vi "Programmed Temperature for Step N.vi"(11 "步骤编号":i32) -> (1 "新的温度消息":string, 3 "待维持的温度":dbl)   [LabVIEW 2015, in "Programmatic Controller.lvclass"]
doc: "给定步骤编号，返回该步骤待维持的温度（数值和字符串）。"
uses:
  Programmatic Controller.lvclass
panel:
  in  "新的待维持温度消息":string="新的待维持温度：%d"
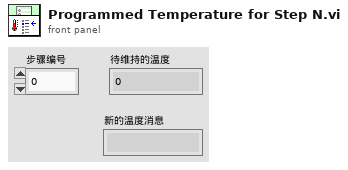
[diagram p1: front panel]
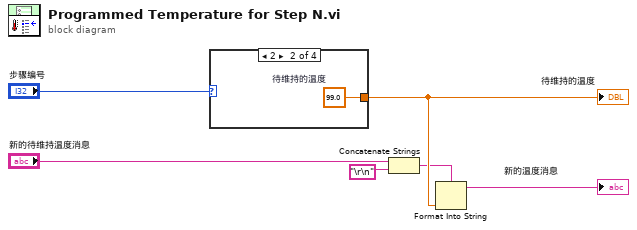
[diagram p0: block diagram]
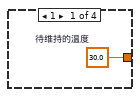
[diagram p2: hidden frame]
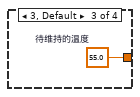
[diagram p3: hidden frame]
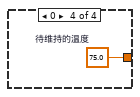
[diagram p4: hidden frame]
diagram:
  n1 = case shown="2" "步骤编号" {
    tunnel: [w7 w8 w9 w10] -> w5
    frame 1 {
      w7 = 30.0  # 待维持的温度
    }
    frame 2 {
      w8 = 99.0  # 待维持的温度
    }
    frame 3, Default {
      w9 = 55.0  # 待维持的温度
    }
    frame 0 {
      w10 = 75.0  # 待维持的温度
    }
  }
  "待维持的温度" <- w5
  n2 = Concatenate Strings("新的待维持温度消息", "\r\n" ("End of Line Constant")) -> (w2:string)
  n3 = Format Into String(format string=w2, w5) -> (resulting string=→"新的温度消息":string)  [unwired: 2 in, 1 out]
